vi "Meas Result Export - Build Report.vi"(8 "error in (no error)":errorcluster, 9 "swp com":string caption="Measurement comment", 10 "append header":bool, 11 "meas":T1 {"src"."cDAQ dds"."channels" min=0 step=1; "bridge"."TWM"."f-list [Hz]" format="%#_6p"; "swp cfg"."f list"."bias" format="%#_3p"; "swp cfg"."f list"."level" format="%#_3p"; "swp cfg"."f list"."fs [Hz]" format="%#_5p"; "swp cfg"."f list"."time [s]" format="%#_3p"; "swp cfg"."f list"."f/fs" format="%#_3p"; "swp cfg"."f list"."periods" format="%#_3f"; "swp cfg"."f list"."f [Hz]" format="%#_5p"}) -> (0 "error out":errorcluster, 3 "report":string[][](array[string]))   [LabVIEW 2020]
doc: "Generates simple results report in form of text matrix."
uses:
  meas session.ctl
  Meas Sweep Config.ctl
  Meas Freq Info.ctl
  meas_swp_mode.ctl
  meas_sweep_flist_mode.ctl
  bridge/Bridge Session.ctl
  bridge/Bridge Type.ctl
  drivers/TWM client/TWM Session.ctl
  drivers/TWM client/TWM parameters.ctl
  drivers/TWM client/Meas Proc QWTB Uncertainty Mode.ctl
  bridge/Bridge Algorithm.ctl
  bridge/Bridge Bias Session.ctl
  bridge/Bridge Bias Type.ctl
  bridge/Bridge Sim Mode.ctl
  source/Source Session.ctl
  source/Source Type.ctl
  drivers/AFG3101C/AFG3101C Session.ctl
  drivers/cDAQ DDS/cDAQ DDS Session.ctl
  drivers/cDAQ DDS/cDAQ DDS Setup.ctl
  drivers/cDAQ DDS/cDAQ DDS Timebase Mode.ctl
  drivers/cDAQ DDS/cDAQ DDS Dither.ctl
  drivers/Fluke 5XXX/top_lev/F5xxx_session.ctl
  drivers/Fluke 5XXX/top_lev/F5xxx_output_mode.ctl
  Meas Results Ref.ctl
  Meas Results.ctl
  bridge/Bridge Frequency Readings Data.ctl
  drivers/TWM client/Meas Proc QWTB Spectrum Data.ctl
  drivers/TWM client/TWM Phase Info.ctl
  dvm/dvm session.ctl
  dvm/dvm type.ctl
  drivers/Fluke 5790A/top_level/F5790 session.ctl
  Meas Results Sweep Data Uncertainty Mode.ctl
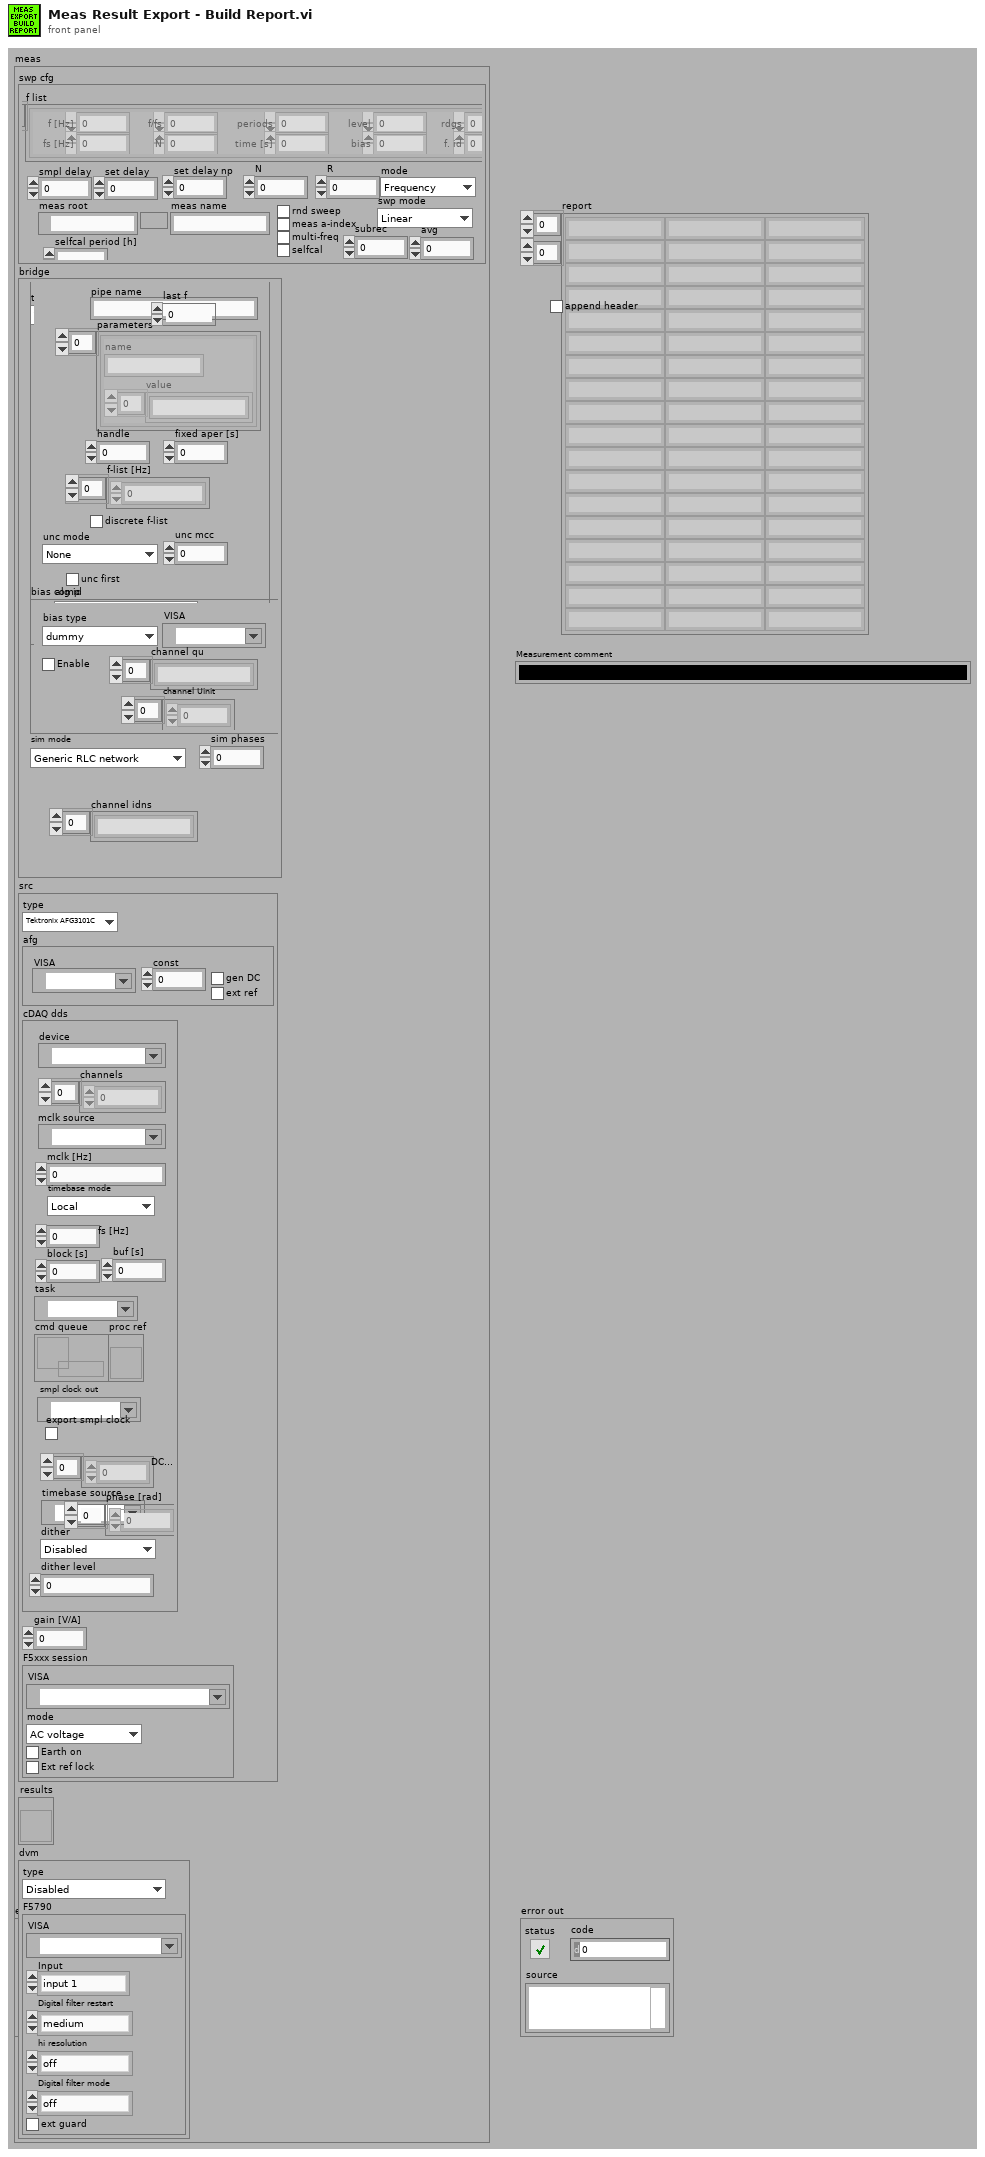
[diagram p1: front panel]
types:
  T1 = typedef "meas session.ctl" = cluster{"swp cfg":T2, "bridge":T6, "src":T15, "results":T23, "dvm":T24}
  T2 = typedef "Meas Sweep Config.ctl" = cluster{"N":i32, "R":i32, "f list":T3[], "smpl delay":dbl, "set delay":dbl, "set delay np":dbl, "meas root":path, "meas name":string, "meas a-index":bool, "rnd sweep":bool, "mode":T4, "swp mode":T5, "avg":i32, "subrec":i32, "multi-freq":bool, "selfcal":bool, "selfcal period [h]":dbl}
  T3 = typedef "Meas Freq Info.ctl" = cluster{"f [Hz]":dbl, "periods":dbl, "f/fs":dbl, "time [s]":dbl, "fs [Hz]":dbl, "N":i32, "level":dbl, "bias":dbl, "rdgs":i32, "f. id":i32}
  T4 = typedef "meas_swp_mode.ctl" = enum16{"Frequency", "Level", "Bias"}
  T5 = typedef "meas_sweep_flist_mode.ctl" = enum16{"Linear", "Log10"}
  T6 = typedef "Bridge Session.ctl" = cluster{"type":T7, "TWM":T8, "last f":dbl, "bias comp":T12, "sim mode":T14, "channel idns":string[], "sim phases":i32}
  T7 = typedef "Bridge Type.ctl" = enum16{"TWM client", "dummy"}
  T8 = typedef "TWM Session.ctl" = cluster{"pipe name":string, "parameters":T9[], "handle":i32, "fixed aper [s]":dbl, "f-list [Hz]":dbl[], "discrete f-list":bool, "unc mode":T10, "unc mcc":i32, "unc first":bool, "alg id":T11}
  T9 = typedef "TWM parameters.ctl" = cluster{"name":string, "value":string[]}
  T10 = typedef "Meas Proc QWTB Uncertainty Mode.ctl" = enum16{"None", "GUF", "Monte Carlo"}
  T11 = typedef "Bridge Algorithm.ctl" = enum16{"TWM-LowZ - Low Z measurement", "TWM-InpZ - Digitizer input Z measurement", "TWM-TIAZ - High Z using TIA"}
  T12 = typedef "Bridge Bias Session.ctl" = cluster{"bias type":T13, "VISA":refnum<visa-resource-name>, "Enable":bool, "channel qu":string[], "channel Uinit":dbl[]}
  T13 = typedef "Bridge Bias Type.ctl" = enum16{"dummy", "CMI LiBbias V1.0"}
  T14 = typedef "Bridge Sim Mode.ctl" = enum16{"Generic RLC network", "Interchannel transfer", "Input impedance"}
  T15 = typedef "Source Session.ctl" = cluster{"type":T16, "afg":T17, "cDAQ dds":T18, "gain [V/A]":dbl, "F5xxx session":T21}
  T16 = typedef "Source Type.ctl" = enum16{"Tektronix AFG3101C", "cDAQ DAC", "Fluke 5xxx", "Agilent 33120A", "dummy"}
  T17 = typedef "AFG3101C Session.ctl" = cluster{"VISA":refnum<visa-resource-name>, "const":dbl, "gen DC":bool, "ext ref":bool}
  T18 = typedef "cDAQ DDS Session.ctl" = cluster{"device":tag, "channels":i32[], "mclk source":tag, "mclk [Hz]":dbl, "fs [Hz]":dbl, "block [s]":dbl, "buf [s]":dbl, "task":refnum<k21>, "cmd queue":refnum<queue>, "proc ref":refnum<vi>, "smpl clock out":tag, "export smpl clock":bool, "DC ofs [V]":dbl[], "timebase source":tag, "timebase mode":T19, "dither":T20, "dither level":dbl, "phase [rad]":dbl[]}
  T19 = typedef "cDAQ DDS Timebase Mode.ctl" = enum16{"Local", "Take from ADC (e.g. NI 9238)", "Other source"}
  T20 = typedef "cDAQ DDS Dither.ctl" = enum16{"Disabled", "Gaussian"}
  T21 = typedef "F5xxx_session.ctl" = cluster{"VISA":refnum<visa-resource-name>, "mode":T22, "Earth on":bool, "Ext ref lock":bool}
  T22 = typedef "F5xxx_output_mode.ctl" = enum16{"AC voltage", "AC current"}
  T23 = typedef "Meas Results Ref.ctl" = refnum<vi>
  T24 = typedef "dvm session.ctl" = cluster{"type":T25, "F5790":T26}
  T25 = typedef "dvm type.ctl" = enum16{"Disabled", "Simulated", "Fluke 5790A"}
  T26 = typedef "F5790 session.ctl" = cluster{"VISA":refnum<visa-resource-name>, "Input":enum16{"input 1", "input 2", "wide-band"}, "Digital filter restart":enum16{"medium", "fine", "coarse"}, "hi resolution":enum16{"off", "on"}, "Digital filter mode":enum16{"off", "fast", "medium", "slow"}, "ext guard":bool}
  T27 = typedef "Meas Results Sweep Data Uncertainty Mode.ctl" = enum16{"ua(y)", "ua(y) (p=95%)", "uc(y) (p=95%)"}
  T28 = typedef "Meas Results.ctl" = cluster{"freqs":T29[][], "locked":bool, "last fid":i32, "modified":bool, "mjr name":string, "mnr name":string, "last spectra":T30[][], "saved?":bool, "TWM phase":T31[], "time start":timestamp, "time stop":timestamp}
  T29 = typedef "Bridge Frequency Readings Data.ctl" = cluster{"Udut":dbl[], "Iref":dbl[], "Udc":dbl[], "Idc":dbl[], "mjr":dbl[], "mnr":dbl[], "mjr_sh":dbl[], "mnr_sh":dbl[], "u(mjr)":dbl[], "u(mnr)":dbl[], "ua2(mjr)":dbl[], "ua2(mnr)":dbl[], "n":i32, "f [Hz]":dbl, "fs [Hz]":dbl, "aperture [s]":dbl, "Udvm":dbl[], "u(Udvm) [V]":dbl}
  T30 = typedef "Meas Proc QWTB Spectrum Data.ctl" = cluster{"x":sgl[], "y":sgl[], "label":string}
  T31 = typedef "TWM Phase Info.ctl" = cluster{"ref chn id (I)":string, "dut chn id (U)":string, "ref chn range [V]":dbl, "dut chn range [V]":dbl, "aperture [s]":dbl, "fs [Hz]":dbl, "ref chn transducer (I)":string, "dut chn transducer (U)":string}
  T32 = typedef "Meas Results Sweep Data.ctl" = cluster{"Udut":dbl[], "Iref":dbl[], "Udc":dbl[], "Idc":dbl[], "mjr":dbl[], "mnr":dbl[], "mjr_sh":dbl[], "mnr_sh":dbl[], "f [Hz]":dbl[], "n [-]":i32[], "fs [Hz]":dbl[], "aperture [s]":dbl[], "Udvm":dbl[]}
  T33 = typedef "Meas Quantity Names.ctl" = cluster{"mjr name":string, "mnr name":string, "mjr unit":string, "mnr unit":string, "mjr full":string, "mnr full":string}
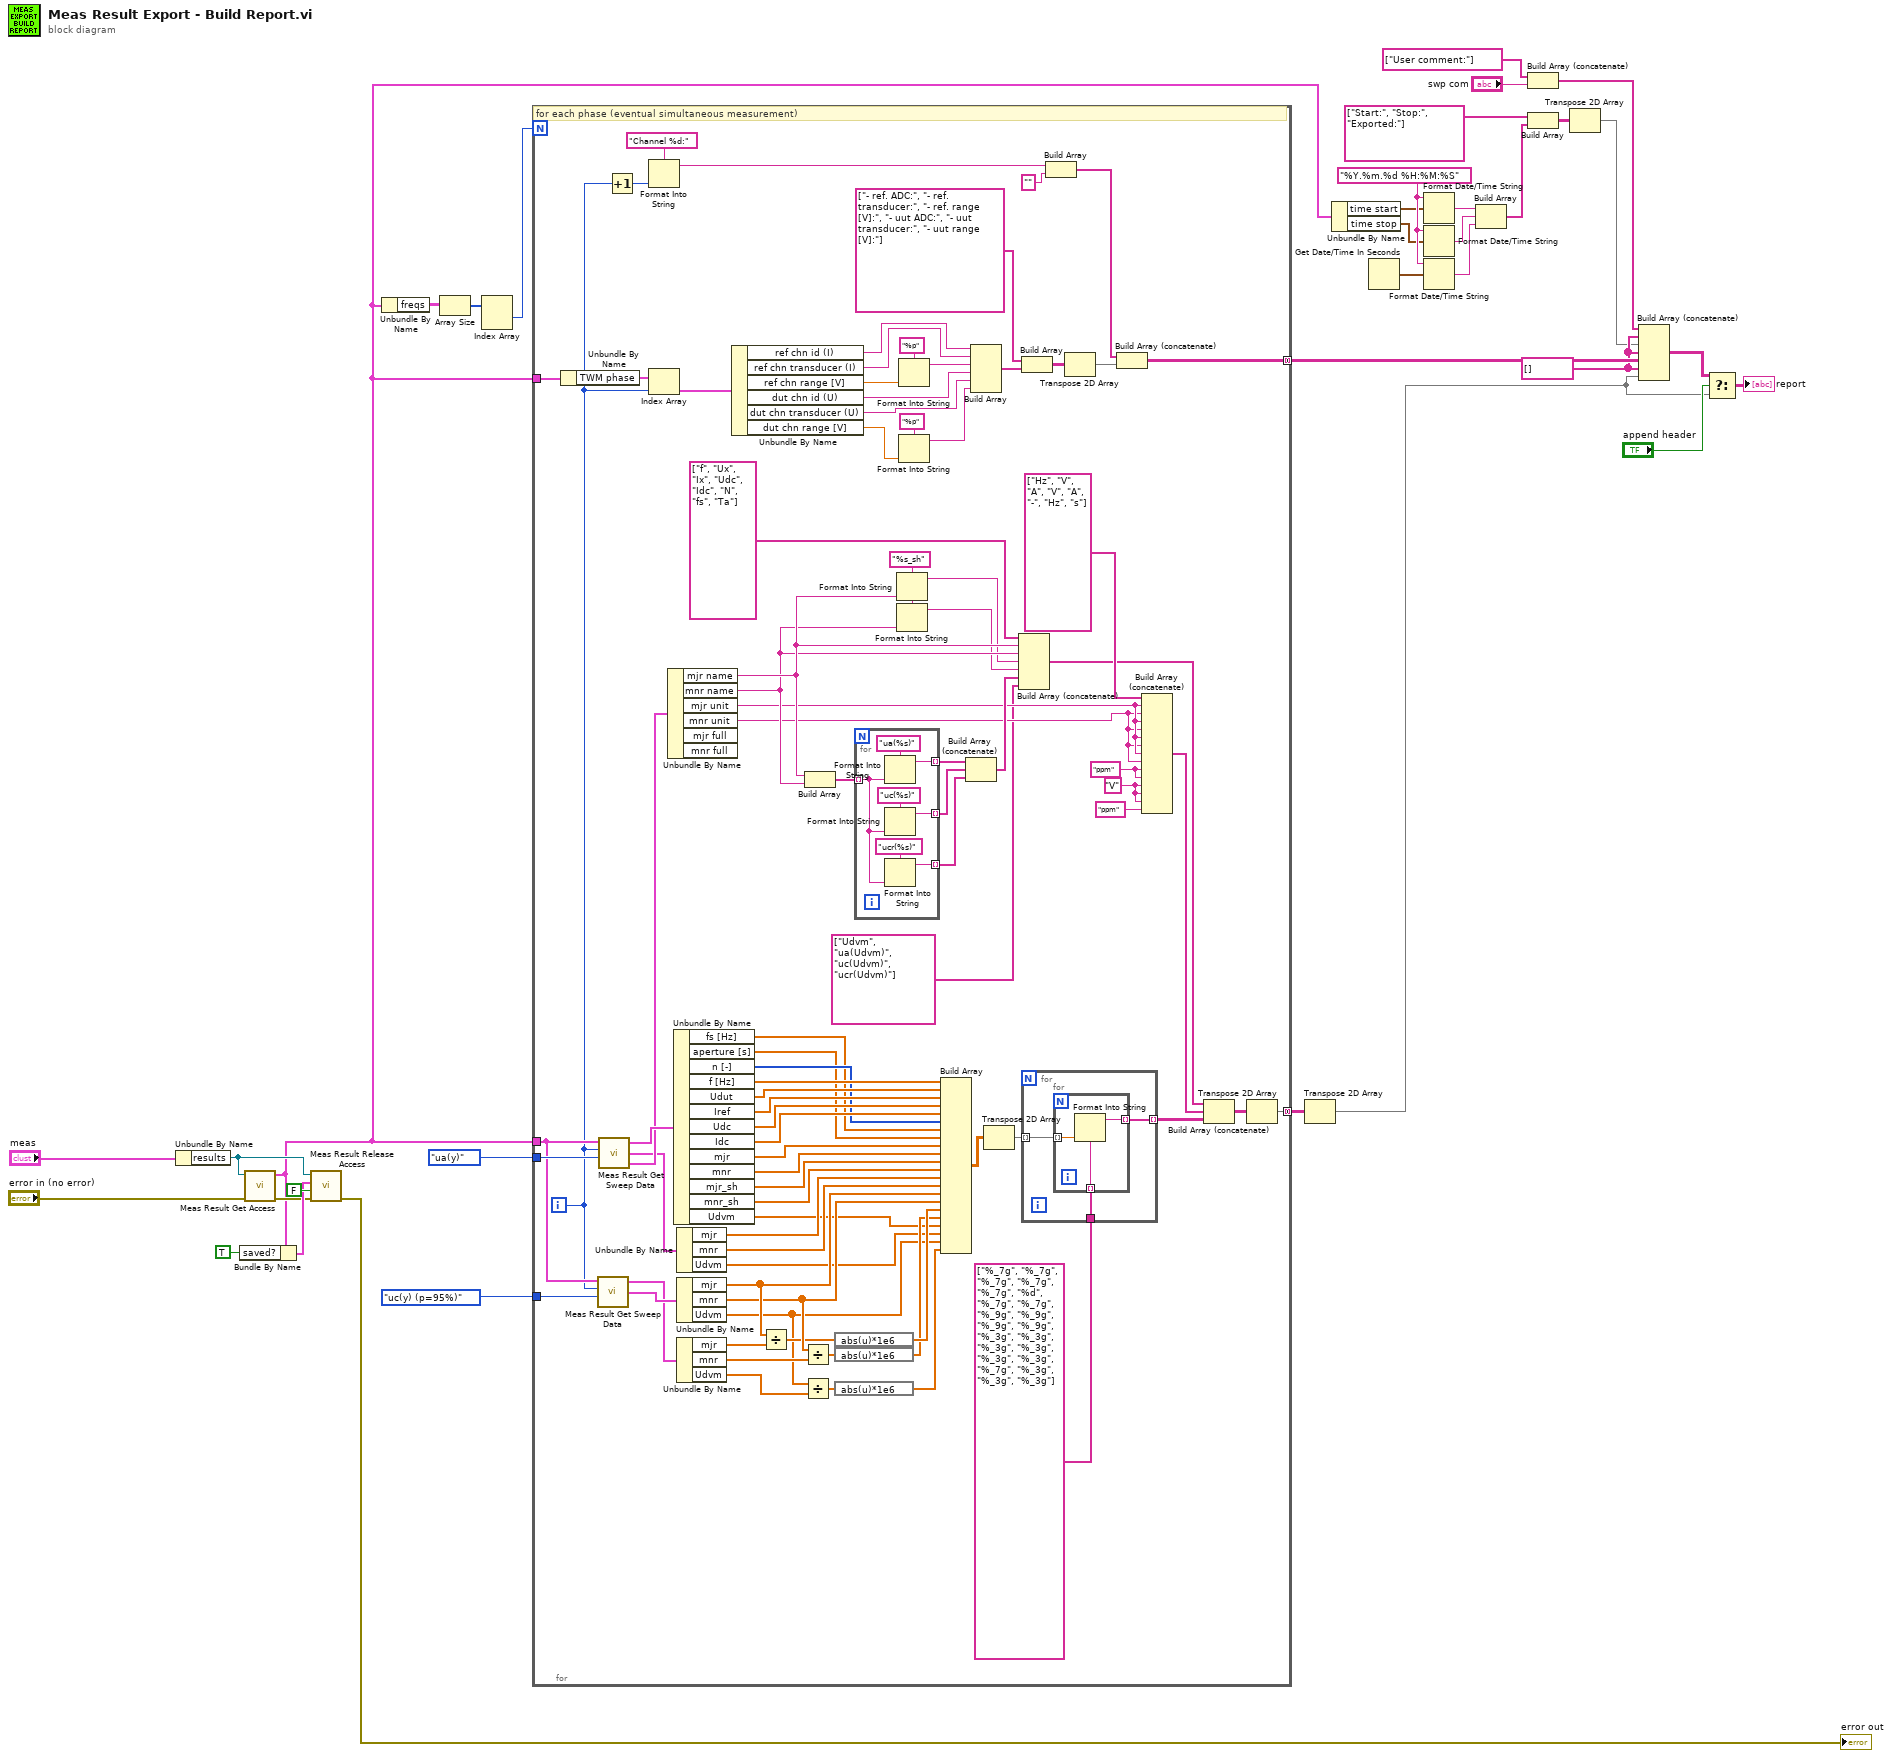
[diagram p0: block diagram]
diagram:
  w12 = string[] [] ("array")
  w10 = "%Y.%m.%d %H:%M:%S" ("format string")
  n1 = Unbundle By Name("meas") -> ("results"=w30:T23)
  n2 = call "Meas Result Get Access.vi"("error in"="error in (no error)", "results ref"=w30) -> ("error out"=w26:errorcluster, "results data"=w5:T28)  [unwired: 8 in]
  n3 = Bundle By Name(cluster=w5, "saved?"=TRUE) -> (w29:T28)
  n4 = call "Meas Result Release Access.vi"("error in"=w26, "Release only (True)"=FALSE, "results data in"=w29, "results ref"=w30) -> ("error out"=→"error out":errorcluster)  [unwired: 7 in]
  n5 = Unbundle By Name(w5) -> ("freqs"=w23:T29[][])
  n6 = Array Size(array=w23) -> (size(s)=w24:i32[])
  n7 = Index Array(array=w24) -> (element #1=w25:i32)  [unwired: 2 in, 1 out]
  n8 = for {
    N: w25 -> [_]
    tunnel: [w72] -> w20 mode=concatenating
    tunnel: Meas_Results_Sweep_Data_Uncertainty_Mode."ua(y)" ("uncertainty mode") -> [w102]
    tunnel: w5 -> [w101]
    tunnel: Meas_Results_Sweep_Data_Uncertainty_Mode."uc(y) (p=95%)" ("uncertainty mode") -> [w100]
    tunnel: w5 -> [w70]
    tunnel: [w47] -> w35 mode=concatenating
    i -> [w66]
    w45 = "V" ("element")
    w74 = "ppm" ("element")
    w90 = "%s_sh" ("format string")
    # "for each phase (eventual simultaneous measurement)"
    n9 = Unbundle By Name(w70) -> ("TWM phase"=w69:T31[])
    n10 = call "Meas Result Get Sweep Data.vi"("uncertainty mode"=w100, "phase index (default: 0)"=w66, "result"=w101) -> ("unc(data)"=w99:T32, "data"=w83:T32)  [unwired: 1 in, 1 out]
    n11 = call "Meas Result Get Sweep Data.vi"("uncertainty mode"=w102, "phase index (default: 0)"=w66, "result"=w101) -> ("quantities"=w120:T33, "unc(data)"=w103:T32, "data"=w121:T32)  [unwired: 1 in]
    n12 = Increment(x=w66) -> (x+1=w65:i32)
    n13 = Format Into String(format string="Channel %d:", w65) -> (resulting string=w64:string)  [unwired: 2 in, 1 out]
    n14 = Index Array(array=w69, index=w66) -> (element=w68:T31)
    n15 = Unbundle By Name(w120) -> ("mjr name"=w89:string, "mnr name"=w88:string, "mjr unit"=w85:string, "mnr unit"=w84:string)  [unwired: 2 out]
    n16 = Unbundle By Name(w121) -> ("fs [Hz]"=w37:dbl[], "aperture [s]"=w36:dbl[], "n [-]"=w71:i32[], "f [Hz]"=w118:dbl[], "Udut"=w117:dbl[], "Iref"=w116:dbl[], "Udc"=w115:dbl[], "Idc"=w114:dbl[], "mjr"=w113:dbl[], "mnr"=w112:dbl[], "mjr_sh"=w92:dbl[], "mnr_sh"=w91:dbl[], "Udvm"=w43:dbl[])
    n17 = Unbundle By Name(w103) -> ("mjr"=w98:dbl[], "mnr"=w97:dbl[], "Udvm"=w42:dbl[])
    n18 = Unbundle By Name(w99) -> ("mjr"=w82:dbl[], "mnr"=w79:dbl[], "Udvm"=w39:dbl[])
    n19 = Unbundle By Name(w83) -> ("mjr"=w81:dbl[], "mnr"=w80:dbl[], "Udvm"=w40:dbl[])
    n20 = Unbundle By Name(w68) -> ("ref chn id (I)"=w56:string, "ref chn transducer (I)"=w57:string, "ref chn range [V]"=w62:dbl, "dut chn id (U)"=w55:string, "dut chn transducer (U)"=w54:string, "dut chn range [V]"=w59:dbl)
    n21 = Divide(x=w82, y=w81) -> (x/y=w77:dbl[])
    n22 = Divide(x=w79, y=w80) -> (x/y=w78:dbl[])
    n23 = Divide(x=w39, y=w40) -> (x/y=w41:dbl[])
    n24 = Build Array(w89, w88) -> (w96:string[])
    n25 = expression code="abs(u)*1e6"(w77) -> (w76:dbl[])
    n26 = expression code="abs(u)*1e6"(w78) -> (w75:dbl[])
    n27 = expression code="abs(u)*1e6"(w41) -> (w38:dbl[])
    n28 = for {
      tunnel: w96 -> [w123] mode=indexing
      tunnel: [w126] -> w95 mode=indexing
      tunnel: [w125] -> w94 mode=indexing
      tunnel: [w122] -> w73 mode=indexing
      n29 = Format Into String(format string="ua(%s)", w123) -> (resulting string=w126:string)  [unwired: 2 in, 1 out]
      n30 = Format Into String(format string="uc(%s)", w123) -> (resulting string=w125:string)  [unwired: 2 in, 1 out]
      n31 = Format Into String(format string="ucr(%s)", w123) -> (resulting string=w122:string)  [unwired: 2 in, 1 out]
    }
    n32 = Format Into String(format string=w90, w89) -> (resulting string=w87:string)  [unwired: 2 in, 1 out]
    n33 = Format Into String(format string=w90, w88) -> (resulting string=w86:string)  [unwired: 2 in, 1 out]
    n34 = Format Into String(format string="%p", w62) -> (resulting string=w58:string)  [unwired: 2 in, 1 out]
    n35 = Format Into String(format string="%p", w59) -> (resulting string=w53:string)  [unwired: 2 in, 1 out]
    n36 = Build Array(w118, w117, w116, w115, w114, w71, w37, w36, w113, w112, w92, w91, w98, w97, w82, w79, w76, w75, w43, w42, w39, w38) -> (w110:dbl[][])
    n37 = Build Array (concatenate)(w95, w94, w73) -> (w93:string[])
    n38 = Build Array(w56, w57, w58, w55, w54, w53) -> (w52:string[])
    n39 = Transpose 2D Array(2D array=w110) -> (transposed array=w109:dbl[][])
    n40 = Build Array (concatenate)(string[] ["f", "Ux", "Ix", "Udc", "Idc", "N", "fs", "Ta"], w89, w88, w87, w86, w93, string[] ["Udvm", "ua(Udvm)", "uc(Udvm)", "ucr(Udvm)"]) -> (w106:string[])
    n41 = Build Array(string[] ["- ref. ADC:", "- ref. transducer:", "- ref. range [V]:", "- uut ADC:", "- uut transducer:", "- uut range [V]:"], w52) -> (w50:string[][])
    n42 = for {
      tunnel: w109 -> [w130] mode=indexing
      tunnel: string[] ["%_7g", "%_7g", "%_7g", "%_7g", "%_7g", "%d", "%_7g", "%_7g", "%_9g", "%_9g", "%_9g", "%_9g", "%_3g", "%_3g", "%_3g", "%_3g", "%_3g", "%_3g", "%_7g", "%_3g", "%_3g", "%_3g"] -> [w131]
      tunnel: [w129] -> w107 mode=indexing
      n43 = for {
        tunnel: w131 -> [w133] mode=indexing
        tunnel: w130 -> [w134] mode=indexing
        tunnel: [w132] -> w129 mode=indexing
        n44 = Format Into String(format string=w133, w134) -> (resulting string=w132:string)  [unwired: 2 in, 1 out]
      }
    }
    n45 = Build Array(w64, "" ("element")) -> (w48:string[])
    n46 = Transpose 2D Array(2D array=w50) -> (transposed array=w49:string[][])
    n47 = Build Array (concatenate)(w48, w49) -> (w47:string[][])
    n48 = Build Array (concatenate)(string[] ["Hz", "V", "A", "V", "A", "-", "Hz", "s"], w85, w84, w85, w84, w85, w84, w85, w84, w74, w74, w45, w45, w45, "ppm" ("element")) -> (w105:string[])
    n49 = Build Array (concatenate)(w106, w105, w107) -> (w104:string[][])
    n50 = Transpose 2D Array(2D array=w104) -> (transposed array=w72:string[][])
  }
  n51 = Transpose 2D Array(2D array=w20) -> (transposed array=w17:string[][])
  n52 = Unbundle By Name(w5) -> ("time start"=w4:timestamp, "time stop"=w3:timestamp)
  n53 = Get Date/Time In Seconds() -> (seconds since 1Jan1904=w11:timestamp)
  n54 = Format Date/Time String(time format string (%c)=w10, seconds (now)=w4) -> (date/time string=w9:string)  [unwired: 1 in]
  n55 = Format Date/Time String(time format string (%c)=w10, seconds (now)=w3) -> (date/time string=w8:string)  [unwired: 1 in]
  n56 = Format Date/Time String(time format string (%c)=w10, seconds (now)=w11) -> (date/time string=w7:string)  [unwired: 1 in]
  n57 = Build Array(w9, w8, w7) -> (w6:string[])
  n58 = Build Array (concatenate)(string[] ["User comment:"], "swp com") -> (w13:string[])
  n59 = Build Array(string[] ["Start:", "Stop:", "Exported:"], w6) -> (w1:string[][])
  n60 = Transpose 2D Array(2D array=w1) -> (transposed array=w2:string[][])
  n61 = Build Array (concatenate)(w13, w12, w2, w12, w35, w12, w17) -> (w19:string[][])
  n62 = Select(t=w19, s="append header", f=w17) -> (s? t:f=→"report":string[][])
